vi "QCP_Open.vi"(11 "Name":string) -> (0 "error out":errorcluster, 3 "QCP_DevRef_Out":T1)   [LabVIEW 2016]
uses:
  <userlib>/836-libraries/System/QCP_V2/QCPSupportCode/QCP_RefNum.ctl
  <userlib>/836-libraries/System/QCP_V2/QCPSupportCode/QCPData.ctl
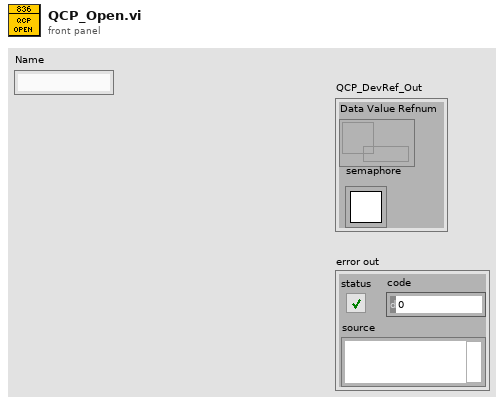
[diagram p1: front panel]
types:
  T1 = typedef "QCP_RefNum.ctl" = cluster{"Data Value Refnum":refnum<data-value>, "semaphore":T2}
  T2 = typedef "Semaphore RefNum" = refnum<k1>
  T3 = typedef "QCPData.ctl" = cluster{"Names":string[], "Values":cluster{"Array":dbl[]}[]}
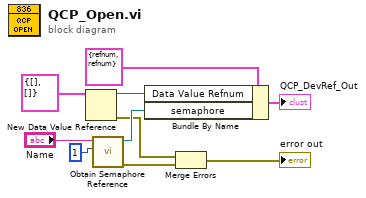
[diagram p0: block diagram]
diagram:
  n1 = New Data Value Reference(data value=T3 {"Names"=[], "Values"=[]} ("QCP Data Ref")) -> (data value reference=w7:refnum<data-value>, error out=w2:errorcluster)  [unwired: 1 in]
  n2 = call <vilib>:"Obtain Semaphore Reference.vi"("size (1)"=1, "name (unnamed)"="Name") -> ("error out"=w3:errorcluster, "semaphore"=w6:T2)  [unwired: 3 in, 1 out]
  n3 = Bundle By Name(cluster=T1 {"Data Value Refnum"=refnum, "semaphore"=refnum} ("QCP_DevRef_Out"), "Data Value Refnum"=w7, "semaphore"=w6) -> (→"QCP_DevRef_Out":T1)
  n4 = Merge Errors(w2, w3) -> (→"error out":errorcluster)
